vi "LH_ObtianArrayFromList.vi"(3 "InputList":refnum<class "ListHead.lvclass">) -> (0 "OutputArray":i32[](array[numeric]), 1 "OutputList":refnum<class "ListHead.lvclass">)   [LabVIEW 2014, in "ListHead.lvclass"]
uses:
  ListHead.lvclass
  ListHead.lvclass/ListHead.ctl
  ListNode.lvclass
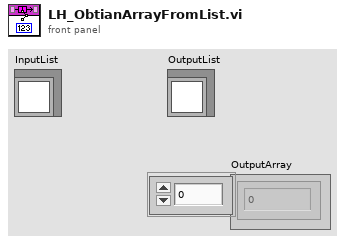
[diagram p1: front panel]
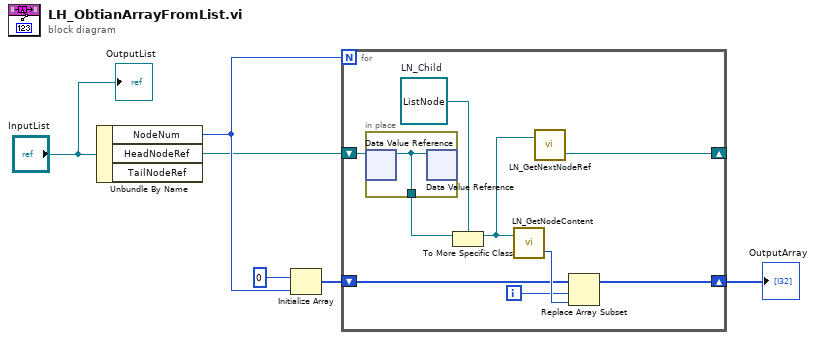
[diagram p0: block diagram]
diagram:
  n1 = Unbundle By Name("InputList") -> ("NodeNum"=w5:u32, "HeadNodeRef"=w2:refnum<data-value>)  [unwired: 1 out]
  n2 = Initialize Array(0, w5) -> (w3:i32[])
  n3 = for {
    N: w5 -> [_]
    shift-right: [w9] -> w1
    shift-left: w3 -> [w11]
    shift-right: [w7] -> _
    shift-left: w2 -> [w15]
    i -> [w10]
    w13 = refnum<class "ListNode.lvclass"> refnum  # LN_Child
    n4 = in-place {
      in-place-border: [w16] -> w14
      n5 = in-place-dvr #1(w15) -> (w16:refnum<class "ListNodeVirtual.lvclass">)  [unwired: 1 out]
      n6 = in-place-dvr #1(w16) -> ()  [unwired: 2 out]
    }
    n7 = To More Specific Class(target class=w13, reference=w14) -> (specific class reference=w8:refnum<class "ListNode.lvclass">)  [unwired: 1 in, 1 out]
    n8 = call "LN_GetNodeContent.vi"("InputNode"=w8) -> ("Content"=w12:i32)  [unwired: 1 in, 1 out]
    n9 = call "LN_GetNextNodeRef.vi"("InputListNode"=w8) -> ("OutputNextNodeRef"=w7:refnum<data-value>)  [unwired: 1 in, 1 out]
    n10 = Replace Array Subset(array=w11, new element=w12, index=w10) -> (w9:i32[])
  }
  "OutputArray" <- w1
  "OutputList" <- "InputList"
